vi "Configure Multi-Point [MP].vi"(5 "sample interval (0.0 s)":dbl format="%.3f", 7 "sample trigger (Immediate)":i32(ring)=1 items=["Immediate"=1, "External"=2, "Software Trigger Function"=3, "Interval"=10, "PXI TRIG0 or VXI TTL0"=111, "PXI TRIG1 or VXI TTL1"=112, "PXI TRIG2 or VXI TTL2"=113, "PXI TRIG3 or VXI TTL3"=114, "PXI TRIG4 or VXI TTL4"=115, "PXI TRIG5 or VXI TTL5"=116, "PXI TRIG6 or VXI TTL6"=117, "PXI TRIG7 or VXI TTL7"=118, "ECL0"=119, "ECL1"=120, "PXI Star"=131, "RTSI 0"=140, "RTSI 1"=141, "RTSI 2"=142, "RTSI 3"=143, "RTSI 4"=144, "RTSI 5"=145, "RTSI 6"=146], 8 "error in (no error)":errorcluster, 9 "sample count (1)":i32=1, 10 "trigger count (1)":i32=1, 11 "CS++DMM in":refnum<class "CS++DMM.lvclass">) -> (0 "error out":errorcluster, 3 "CS++DMM out":refnum<class "CS++DMM.lvclass">)   [LabVIEW 2013, in "CS++DMM.lvlib" / "CS++DMM.lvclass"]
doc: "This VI configures the properties that affect multi-point measurements. These properties are the trigger count, sample count, sample trigger and sample interval.\n\nNote:\n\n(1) This VI is part of the IviDmmMultiPoint [MP] extension group."
uses:
  CS++DMM.lvclass
  CSPP_Core/Classes/CS++ProcessVariables/ProcessVariable/PV.lvclass
  PV-Enum.ctl
  CS++DMM.lvclass/CS++DMM.ctl
  CSPP_Core/Classes/CS++ProcessVariables/PVConnection/PVConnection.lvclass
  CSPP_Core/Classes/CS++ProcessVariables/ProcessVariable/PV.lvclass/PV.ctl
  CSPP_Core/Classes/CS++ProcessVariables/ProcessVariable/Write Data.vi
  CSPP_Core/Classes/CS++ProcessVariables/ProcessVariable/Write Timestamp.vi
  CSPP_Core/Classes/CS++ProcessVariables/ProcessVariable/Write Quality.vi
  CSPP_Core/Classes/CS++ProcessVariables/ProcessVariable/Write status.vi
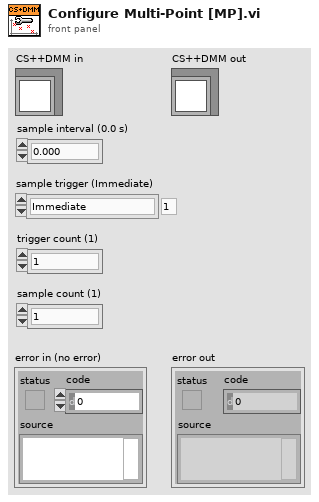
[diagram p1: front panel]
types:
  T1 = typedef "CS++DMM.lvlib/CS++DMM.lvclass/PV-Enum.ctl" = enum16{"AbsoluteResolution", "ACMaxFrequency", "ACMinFrequency", "ActualRange", "Alpha", "ApertureTime", "FixedReferenceJunction", "FrequencyVoltageRange", "PowerLineFrequency", "Range", "Reading", "Resistance", "SampleInterval", "TriggerDelay", "ApertureTimeUnit", "AutoZeroMode", "MeasCompleteDestination", "MeasurementFunction", "ReferenceJunctionType", "SampleCount", "SampleTrigger", "ThermocoupleType", "TranducerType", "TriggerCount", "TriggerSlope", "TriggerSource", "MPReading", "IsOverRange"}
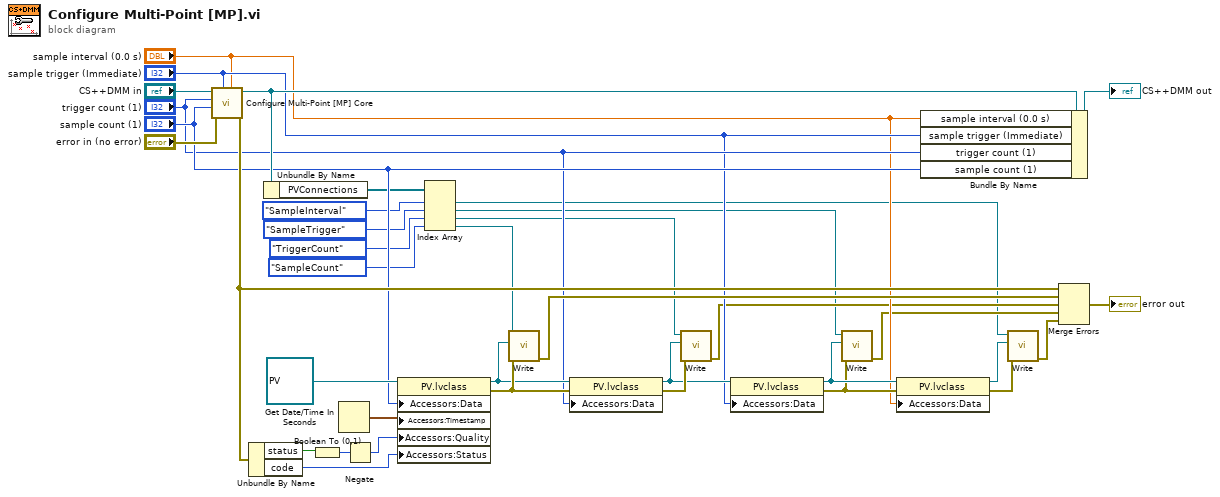
[diagram p0: block diagram]
diagram:
  n1 = call-dynamic "Configure Multi-Point [MP] Core.vi"("sample interval (0.0 s)"="sample interval (0.0 s)", "sample trigger (Immediate)"="sample trigger (Immediate)", "error in (no error)"="error in (no error)", "sample count (1)"="sample count (1)", "trigger count (1)"="trigger count (1)", "CS++DMM in"="CS++DMM in") -> ("error out"=w27:errorcluster, "CS++DMM out"=w26:refnum<class "CS++DMM.lvclass">)  [unwired: 4 in]
  n2 = Unbundle By Name(w27) -> ("status"=w36:bool, "code"=w33:i32)
  n3 = Unbundle By Name(w26) -> ("PVConnections"=w12:refnum<class "PVConnection.lvclass">[])
  n4 = Boolean To (0,1)(Boolean=w36) -> (0, 1=w35:i16)
  n5 = Get Date/Time In Seconds() -> (seconds since 1Jan1904=w32:timestamp)
  n6 = Negate(x=w35) -> (-x=w34:i16)
  n7 = property class="PV.lvclass"(reference=refnum<class "PV.lvclass"> refnum ("CS++ProcessVariables.lvlib:PV.lvclass"), "Accessors:Data"="sample count (1)", "Accessors:Timestamp"=w32, "Accessors:Quality"=w34, "Accessors:Status"=w33) -> (reference out=w21:refnum<class "PV.lvclass">, error out=w22:errorcluster)  [unwired: 1 in]
  n8 = Index Array(array=w12, index #1=PV-Enum."SampleInterval" ("PV-Enum"), index #2=PV-Enum."SampleTrigger" ("PV-Enum"), index #3=PV-Enum."TriggerCount" ("PV-Enum"), index #4=PV-Enum."SampleCount" ("PV-Enum")) -> (element #1=w8:refnum<class "PVConnection.lvclass">, element #2=w5:refnum<class "PVConnection.lvclass">, element #3=w3:refnum<class "PVConnection.lvclass">, element #4=w1:refnum<class "PVConnection.lvclass">)
  n9 = call-dynamic "Write.vi"("error in (no error)"=w22, "PV"=w21, "PVConnection in"=w1) -> ("error out"=w31:errorcluster)  [unwired: 7 in, 1 out]
  n10 = property class="PV.lvclass"(reference=w21, error in=w22, "Accessors:Data"="trigger count (1)") -> (reference out=w19:refnum<class "PV.lvclass">, error out=w23:errorcluster)
  n11 = call-dynamic "Write.vi"("error in (no error)"=w23, "PV"=w19, "PVConnection in"=w3) -> ("error out"=w11:errorcluster)  [unwired: 7 in, 1 out]
  n12 = property class="PV.lvclass"(reference=w19, "Accessors:Data"="sample trigger (Immediate)") -> (reference out=w15:refnum<class "PV.lvclass">, error out=w14:errorcluster)  [unwired: 1 in]
  n13 = call-dynamic "Write.vi"("error in (no error)"=w14, "PV"=w15, "PVConnection in"=w5) -> ("error out"=w10:errorcluster)  [unwired: 7 in, 1 out]
  n14 = property class="PV.lvclass"(reference=w15, error in=w14, "Accessors:Data"="sample interval (0.0 s)") -> (reference out=w16:refnum<class "PV.lvclass">, error out=w17:errorcluster)
  n15 = Bundle By Name(cluster=w26, "sample interval (0.0 s)"="sample interval (0.0 s)", "sample trigger (Immediate)"="sample trigger (Immediate)", "trigger count (1)"="trigger count (1)", "sample count (1)"="sample count (1)") -> (→"CS++DMM out":refnum<class "CS++DMM.lvclass">)
  n16 = call-dynamic "Write.vi"("error in (no error)"=w17, "PV"=w16, "PVConnection in"=w8) -> ("error out"=w9:errorcluster)  [unwired: 7 in, 1 out]
  n17 = Merge Errors(w27, w31, w11, w10, w9) -> (→"error out":errorcluster)
